vi "CAN Get Msg.vi"(9 "pCanGetMsg":T1, 10 "CANIndex":u8, 11 "DevHandle":i32) -> (1 "pCanGetMsg out":T1, 3 "function return":i32)   [LabVIEW 2010, in "usb2can.lvlib"]
doc: "int WINAPI CAN_GetMsg(int DevHandle, unsigned char CANIndex, CAN_MSG *pCanGetMsg);"
uses:
  usb2can.lvlib
  USB2XXX/trunk/USB2XXX/USB2XXX/vs2019/Release/USB2XXX.dll
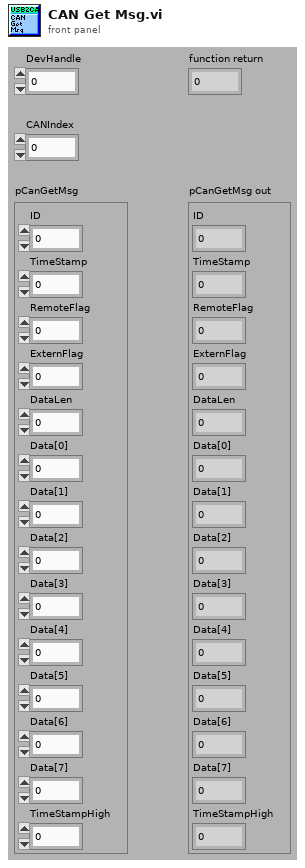
[diagram p1: front panel]
types:
  T1 = cluster{"ID":u32, "TimeStamp":u32, "RemoteFlag":u8, "ExternFlag":u8, "DataLen":u8, "Data[0]":u8, "Data[1]":u8, "Data[2]":u8, "Data[3]":u8, "Data[4]":u8, "Data[5]":u8, "Data[6]":u8, "Data[7]":u8, "TimeStampHigh":u8}
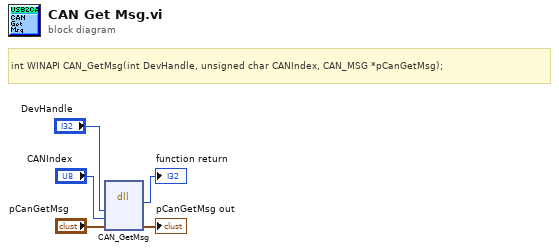
[diagram p0: block diagram]
diagram:
  # "int WINAPI CAN_GetMsg(int DevHandle, unsigned char CANIndex, CAN_MSG *pCanGetMsg);"
  n1 = dll-call lib="E:/Projects/USB2XXX/trunk/USB2XXX/USB2XXX/vs2019/Release/USB2XXX.*" fn="CAN_GetMsg"("DevHandle"="DevHandle", "CANIndex"="CANIndex", "pCanGetMsg"="pCanGetMsg") -> (→"function return":i32, "pCanGetMsg"=→"pCanGetMsg out":T1)  [unwired: 5 in, 2 out]
